vi "Active Task FGV.vi"(7 "Write/Read":enum16{"Write", "Read"}(ring)=enum."Read", 8 "error in":errorcluster, 11 "Activate Task":T1) -> (0 "error out":errorcluster, 3 "Activate Task 2":T1)   [LabVIEW 2022 SP3]
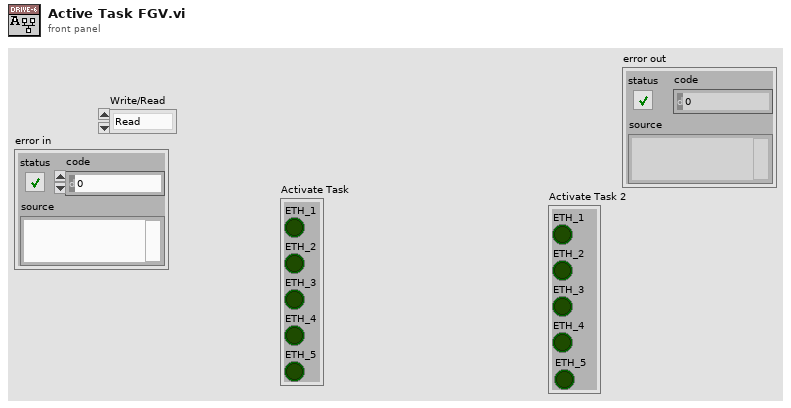
[diagram p1: front panel]
types:
  T1 = cluster{"ETH_1":bool, "ETH_2":bool, "ETH_3":bool, "ETH_4":bool, "ETH_5":bool}
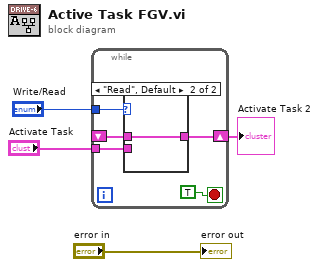
[diagram p0: block diagram]
diagram:
  n1 = while {
    tunnel: "Write/Read" -> [w9]
    tunnel: "Activate Task" -> [w7]
    shift-right: [w6] -> w1
    shift-left: _ -> [w5]
    stop <- TRUE stop-if-true
    n2 = case shown="\"Read\", Default" w9 {
      tunnel: w7 -> [w10 _]
      tunnel: [w10 w11] -> w6
      tunnel: w5 -> [_ w11]
      frame "Write" {
      }
      frame "Read", Default {
      }
    }
  }
  "Activate Task 2" <- w1
  "error out" <- "error in"
